vi "Read connection.vi"(8 "error in (no error)":errorcluster, 11 "RP Communicator in":refnum<class "RP Communicator.lvclass">) -> (0 "error out":errorcluster, 2 "connection":refnum<k5>, 3 "RP Communicator out":refnum<class "RP Communicator.lvclass">)   [LabVIEW 2015, in "RP Communicator.lvclass"]
uses:
  RP Communicator.lvclass
  RP Communicator.lvclass/RP Communicator.ctl
panel:
  out "NaN/Path/Refnum?":bool
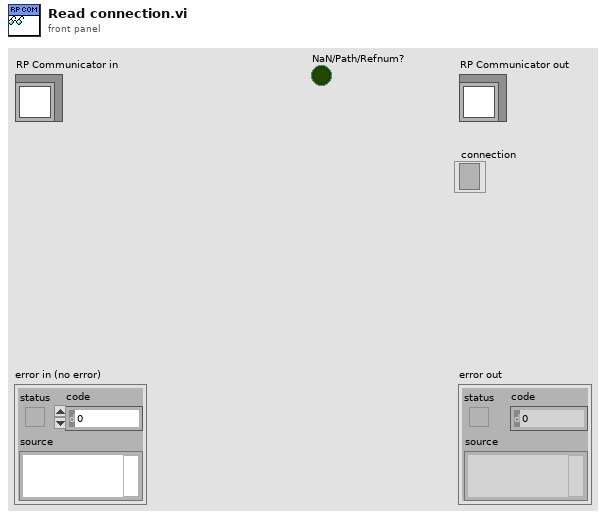
[diagram p1: front panel]
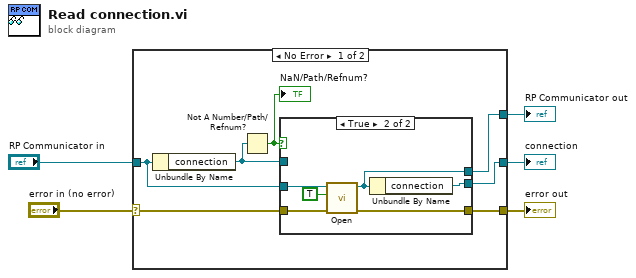
[diagram p0: block diagram]
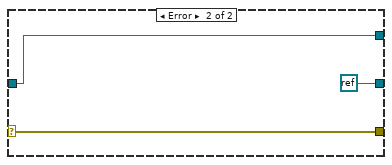
[diagram p3: hidden frame]
diagram:
  n1 = case shown="No Error" "error in (no error)" {
    selector: "error in (no error)" -> [w9 w23]
    tunnel: [w8 w23] -> w4
    tunnel: [w10 w24] -> w2
    tunnel: "RP Communicator in" -> [w11 w24]
    tunnel: [w6 refnum<k0> refnum] -> w1
    frame No Error {
      n2 = Unbundle By Name(w11) -> ("connection"=w7:refnum<k5>)
      n3 = Not A Number/Path/Refnum?(number/path/refnum=w7) -> (NaN/Path/Refnum?=w12:bool)
      "NaN/Path/Refnum?" <- w12
      n4 = case shown="True" w12 {
        tunnel: w11 -> [w15 w19]
        tunnel: [w15 w18] -> w10
        tunnel: w9 -> [w14 w21]
        tunnel: [w14 w20] -> w8
        tunnel: w7 -> [w13 _]
        tunnel: [w13 w17] -> w6
        frame False {
        }
        frame True {
          n5 = call-dynamic "Open.vi"("error in (no error)"=w21, "Send \"Connect client\""=TRUE ("Send \"Connect client\""), "RP Communicator in"=w19) -> ("error out"=w20:errorcluster, "RP Communicator out"=w18:refnum<class "RP Communicator.lvclass">)  [unwired: 7 in]
          n6 = Unbundle By Name(w18) -> ("connection"=w17:refnum<k5>)
        }
      }
    }
    frame Error {
    }
  }
  "error out" <- w4
  "RP Communicator out" <- w2
  "connection" <- w1
